vi "Application UI.vi"() -> ()   [LabVIEW 2023, in "User Interface.lvlib"]
uses:
  User Interface.lvlib
  Controls/main consumer cluster.ctl
  File Classes/File/File.lvclass
  Controls/configuration cluster.ctl
  File Classes/Controls/exif data cluster.ctl
  File Classes/Controls/rename type enum.ctl
  Controls/app operation state enum.ctl
  Controls/main producer cluster.ctl
  <vilib>/Utility/error.llb/Trim Whitespace One-Sided.vi
  EXIF Modifier/EXIF UI.vi
  EXIF Modifier/EXIF Modifier.lvlib
  File Classes/File Classes.lvlib
panel:
  in  "Temp":bool
  in  "Mode":enum16{"Copy (Default)", "Move", "Rename"}(ring)
  in  "File Name Format":T1(ring)
  in  "Event Name":string
  in  "Jpg?":bool
  in  "Exclude Folder":string
  in  "Add Scanner":string
  in  "Delete Folder":bool
  in  "Add Folder":bool
  in  "Delete Scan":bool
  in  "Add Scan":bool
  in  "Exclude":i32(listbox)=-1
  in  "Scanner":i32(listbox)=-1
  in  "Log?":bool=TRUE
  in  "Pause":bool
  in  "Stop":bool
  in  "Start":bool
  out "String":string
  out "Slide":dbl(slide) scale=0.0..100.0
  in  "Destination Path":path
  in  "Source Path":path
  out "Status":string="Application started. Waiting for user input ....."
  in  "Producer Cluster In":T2
  in  "Consumer Cluster in":T3={"This VI Ref"=refnum, "Test VI"=refnum, "Q Ref"=refnum, "UE"=refnum, "Data"=variant, "Timeout"=-1, "Path List[]"=[], "Status"="", "Counter"=0, "Config"={"Source Path"=path "", "Dest Path"=path "", "Log Path"=path "", "Move?"=FALSE, "Log?"=FALSE, "Scanners"=[], "Excude Folders"=[], "Jpg?"=FALSE, "Default path"=path "", "Extended?"=FALSE, "Mode"=enum."Move", "Temp"=FALSE}, "Total"=0, "Config Path"=path "", "exif info"={"Make"="Canon\u0000", "Model"="Canon PowerShot A495\u0000", "Orientation"=0, "Date"=timestamp(0 s since 1904-01-01), "Width"=0, "Height"=0, "Square?"=FALSE, "File Name"="Canon\u0000", "Extension"="Canon\u0000", "Valid?"=FALSE, "Path"=path "", "size"=0, "No Ext?"=FALSE, "prefix?"=FALSE, "Tag"="", "Name Type"=enum."Event Sufix", "Projection Type"="Canon\u0000"}, "app operation"=enum."Start", "Log Ref"=refnum, "Start Time"=0.0, "Pause Time"=0.0, "Argument?"=FALSE, "Argument path"=path "", "Identical"=FALSE, "File.lvclass"=refnum}
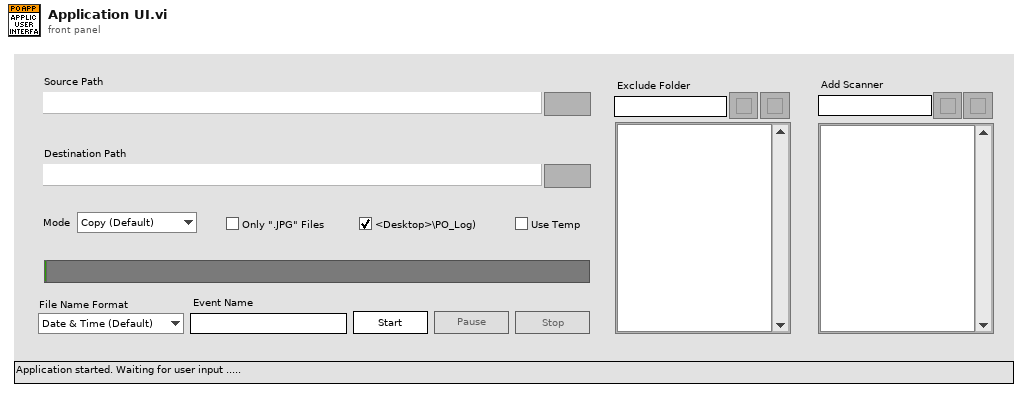
[diagram p1: front panel]
types:
  T1 = enum16{"Date & Time (Default)", "Model Sufix", "Event Sufix", "Model & Event Sufix"}
  T2 = typedef "User Interface.lvlib/main producer cluster.ctl" = cluster{"Q Ref":refnum<queue>, "menu ref":refnum<k9>, "Item Tag":string, "Is EXE?":bool, "This VI Ref":refnum<vi>, "States To Execute":string[]}
  T3 = typedef "User Interface.lvlib/main consumer cluster.ctl" = cluster{"This VI Ref":refnum<vi>, "Test VI":refnum<vi>, "Q Ref":refnum<queue>, "UE":refnum<event-registration>, "Data":variant, "Timeout":i32, "Path List[]":path[], "Status":string, "Counter":i32, "Config":T4, "Total":i32, "Config Path":path, "exif info":T5, "app operation":T7, "Log Ref":refnum<file>, "Start Time":dbl, "Pause Time":dbl, "Argument?":bool, "Argument path":path, "Identical":bool, "File.lvclass":refnum<class "File.lvclass">}
  T4 = typedef "User Interface.lvlib/configuration cluster.ctl" = cluster{"Source Path":path, "Dest Path":path, "Log Path":path, "Move?":bool, "Log?":bool, "Scanners":string[], "Excude Folders":string[], "Jpg?":bool, "Default path":path, "Extended?":bool, "Mode":enum16{"Copy (Default)", "Move", "Rename"}, "Temp":bool}
  T5 = typedef "File Classes.lvlib/exif data cluster.ctl" = cluster{"Make":string, "Model":string, "Orientation":u16, "Date":timestamp, "Width":u16, "Height":u16, "Square?":bool, "File Name":string, "Extension":string, "Valid?":bool, "Path":path, "size":i64, "No Ext?":bool, "prefix?":bool, "Tag":string, "Name Type":T6, "Projection Type":string}
  T6 = typedef "File Classes.lvlib/rename type enum.ctl" = enum16{"Date & Time (Default)", "Model Sufix", "Event Sufix", "Model & Event Sufix"}
  T7 = typedef "User Interface.lvlib/app operation state enum.ctl" = enum16{"Start", "Stop", "Pause", "Resume"}
  T8 = enum32{"invalid app kind", "Development System", "Run Time System", "Student Edition", "Embedded LabVIEW", "Evaluation", "Custom"}
  T9 = enum8{"Enabled", "Disabled", "Disabled and Grayed Out"}
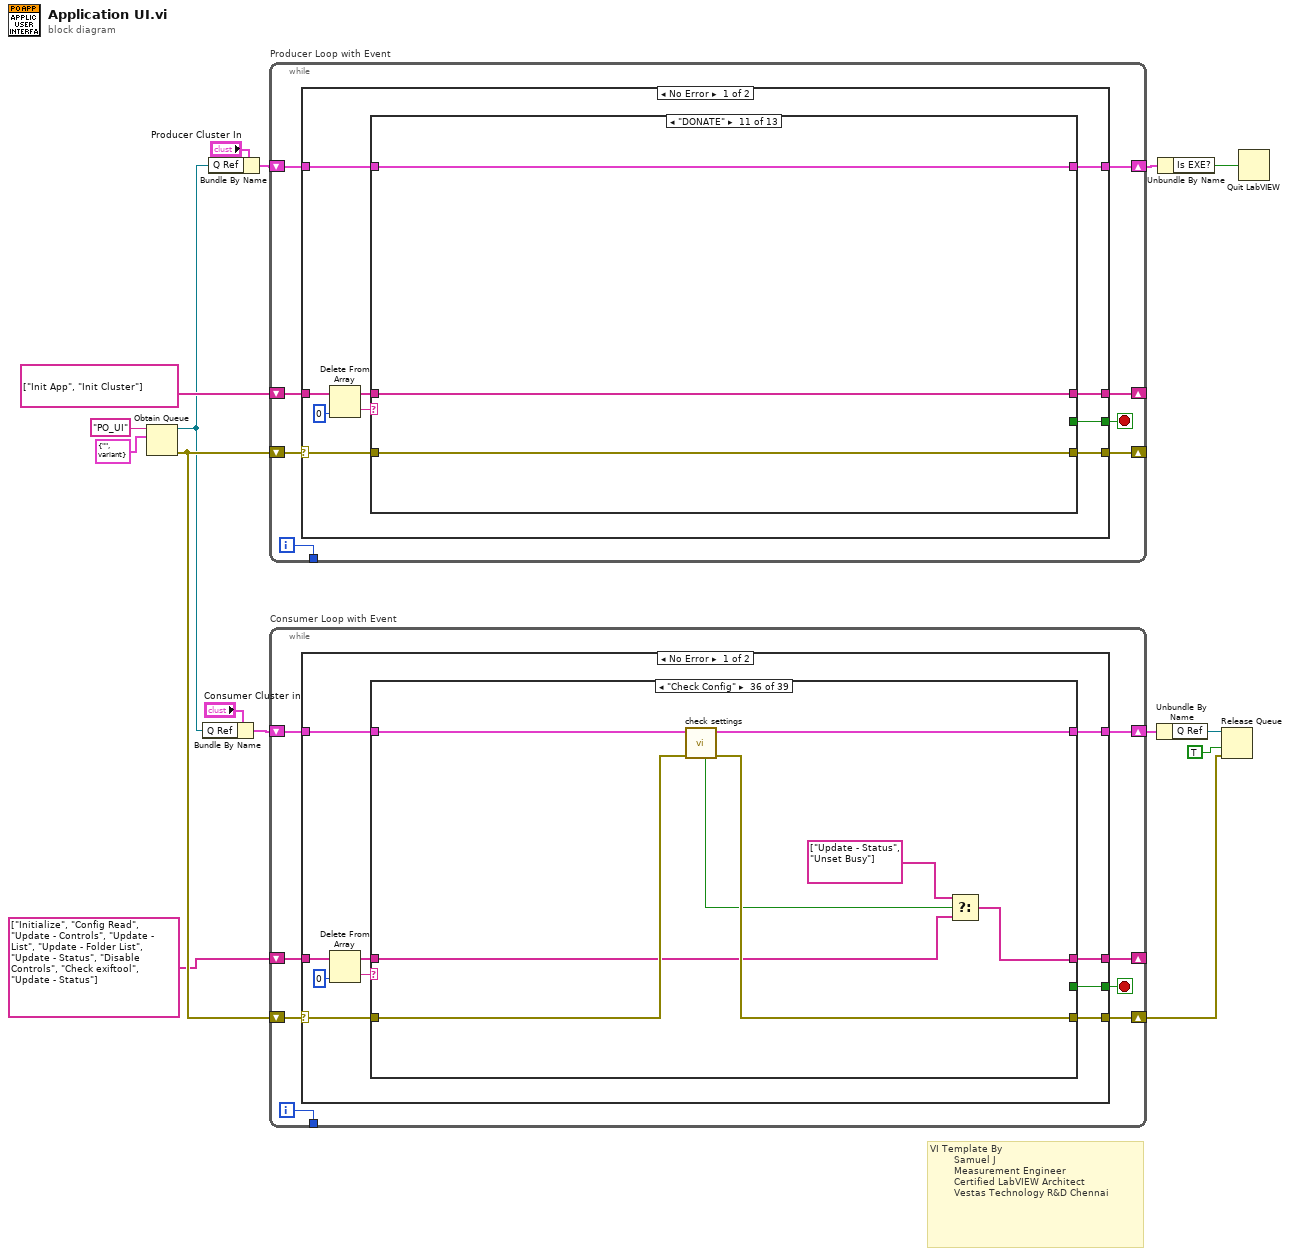
[diagram p0: block diagram]
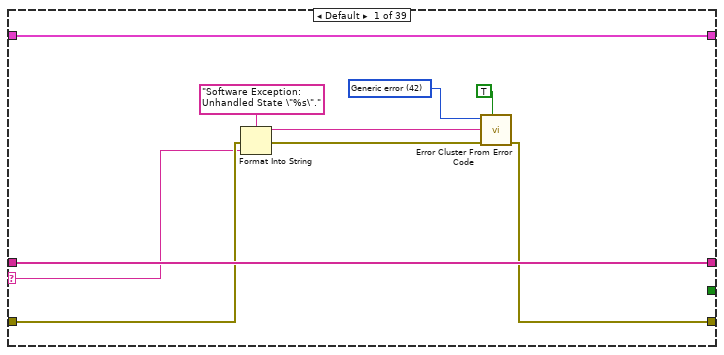
[diagram p2: hidden frame]
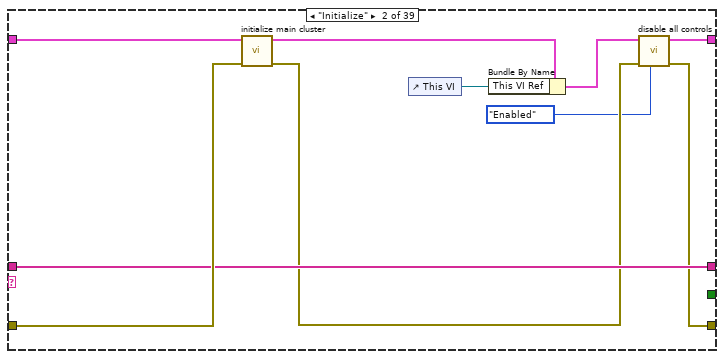
[diagram p3: hidden frame]
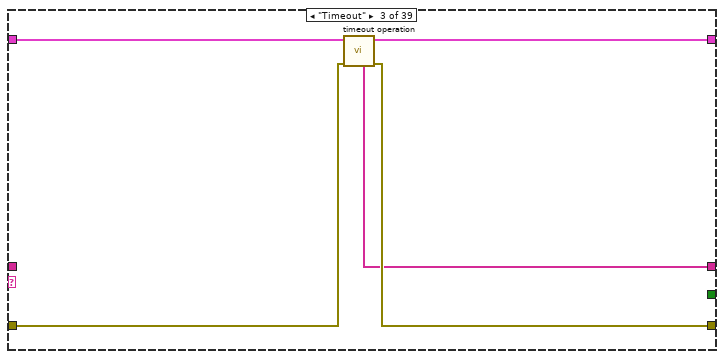
[diagram p4: hidden frame]
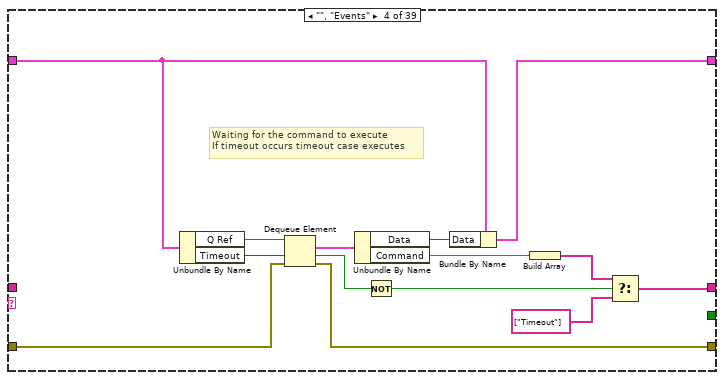
[diagram p5: hidden frame]
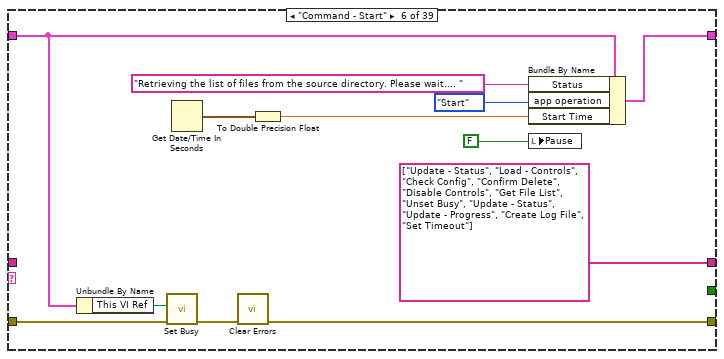
[diagram p7: hidden frame]
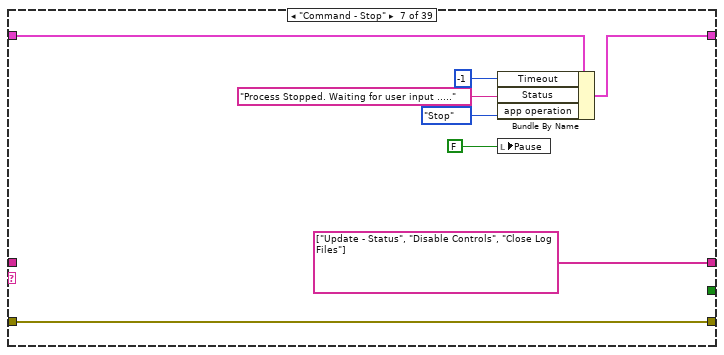
[diagram p8: hidden frame]
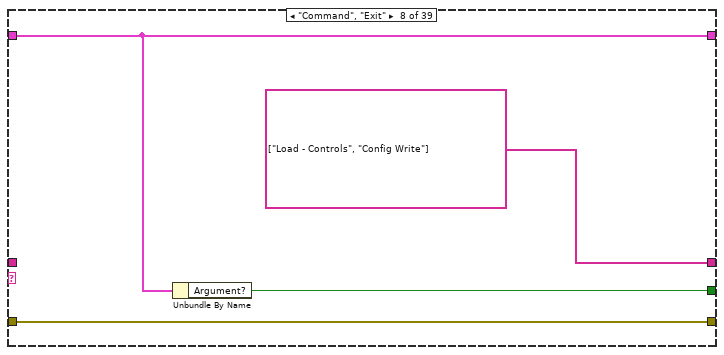
[diagram p9: hidden frame]
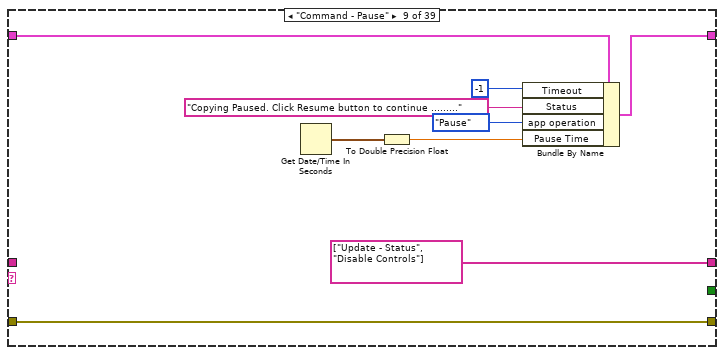
[diagram p10: hidden frame]
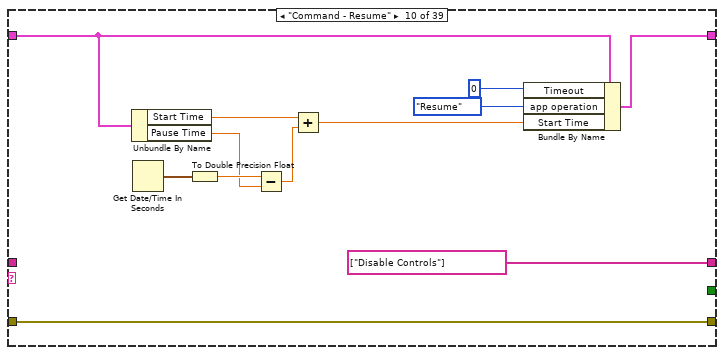
[diagram p11: hidden frame]
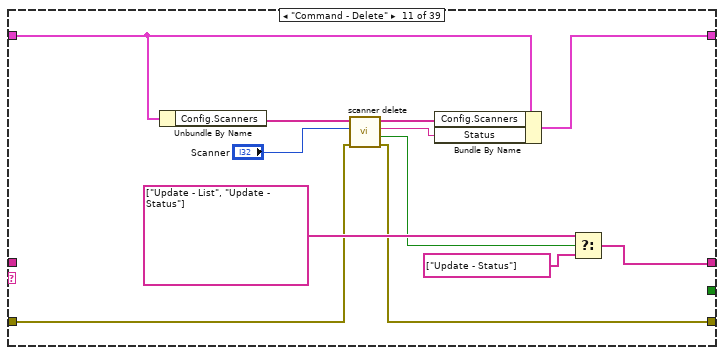
[diagram p12: hidden frame]
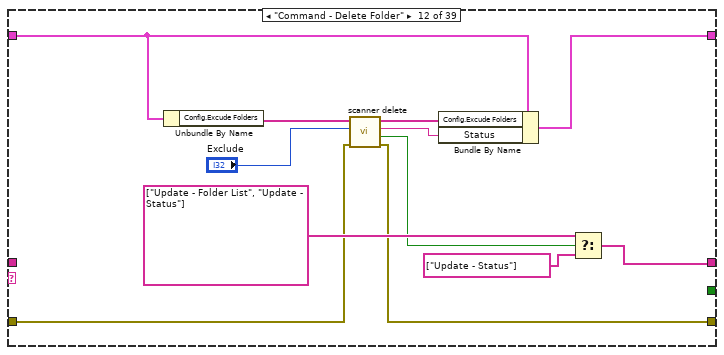
[diagram p13: hidden frame]
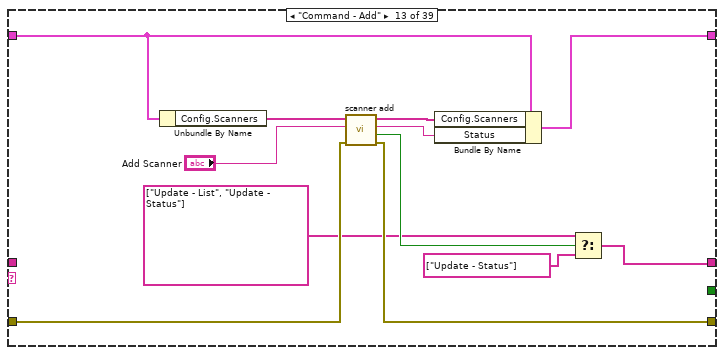
[diagram p14: hidden frame]
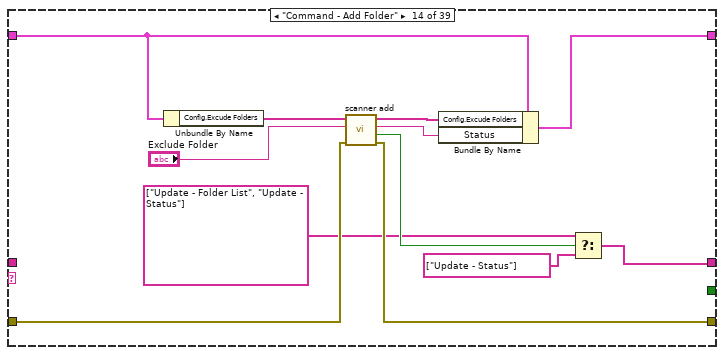
[diagram p15: hidden frame]
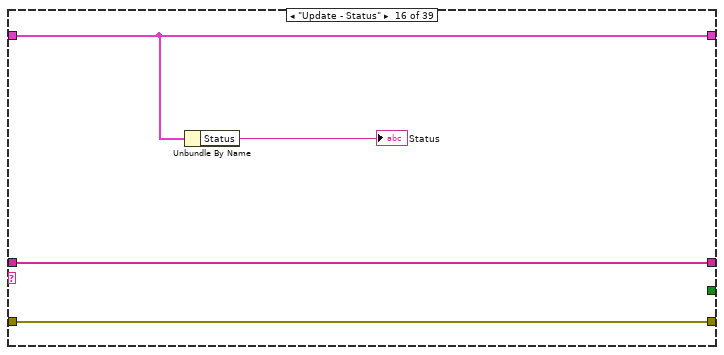
[diagram p17: hidden frame]
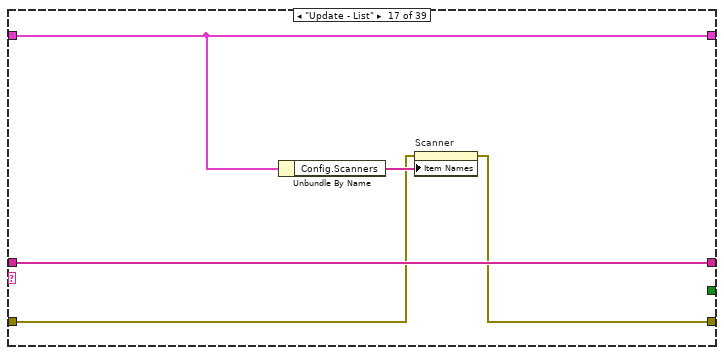
[diagram p18: hidden frame]
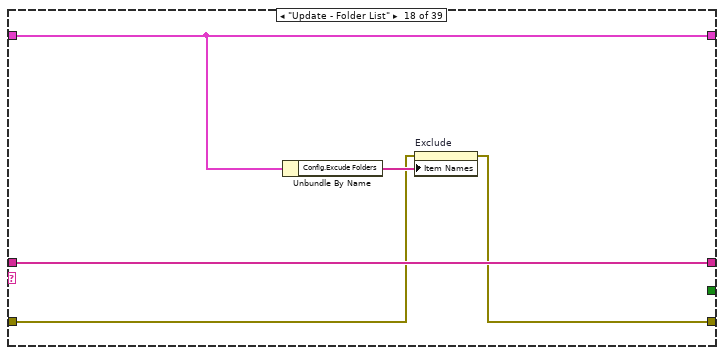
[diagram p19: hidden frame]
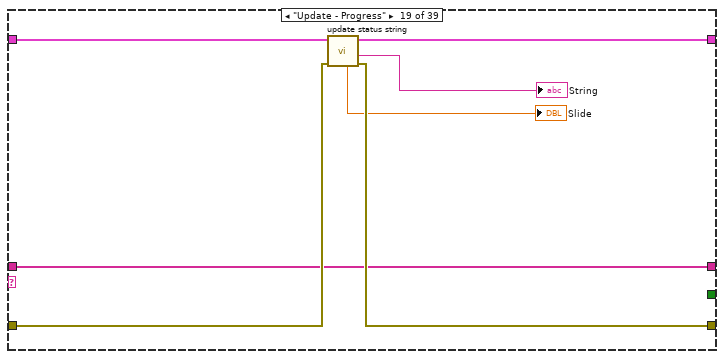
[diagram p20: hidden frame]
diagram:
  # "VI Template By\n        Samuel J\n        Measurement Engineer\n        Certified LabVIEW Architect\n        Vestas Technology R&D Chennai"
  n1 = Obtain Queue(name (unnamed)="PO_UI", element data type=cluster{"Command":string, "Data":variant} {"Command"="", "Data"=variant} ("Data Cluster")) -> (queue out=w12:refnum<queue>, error out=w13:errorcluster)  [unwired: 3 in, 1 out]
  n2 = Bundle By Name(cluster="Consumer Cluster in", "Q Ref"=w12) -> (w14:T3)
  n3 = Bundle By Name(cluster="Producer Cluster In", "Q Ref"=w12) -> (w7:T2)
  n4 = while "Producer Loop with Event" {
    shift-right: [w23] -> _
    shift-left: w13 -> [w24]
    shift-right: [w20] -> _
    shift-left: string[] ["Init App", "Init Cluster"] ("appended array") -> [w21]
    shift-right: [w18] -> w8
    shift-left: w7 -> [w19]
    tunnel: [w17] -> _
    i -> [w17]
    stop <- w22 stop-if-true
    n5 = case shown="No Error" w24 {
      selector: w24 -> [w34 w207]
      tunnel: [w33 w211] -> w23
      tunnel: [w32 FALSE] -> w22
      tunnel: w21 -> [w31 _]
      tunnel: [w27 string[] []] -> w20
      tunnel: w19 -> [w26 w206]
      tunnel: [w25 w206] -> w18
      frame No Error {
        n6 = Delete From Array(array=w31, index=0) -> (deleted portion=w29:string, array with subset deleted=w28:string[])  [unwired: 1 in]
        n7 = case shown="\"DONATE\"" w29 {
          selector: w29 -> [w37 _ _ _ _ _ _ _ _ _ _ _ _]
          tunnel: w34 -> [w39 w56 w65 w70 w86 w162 w167 w177 w185 w189 w192 w195 w199]
          tunnel: [w38 w49 w65 w68 w85 w162 w167 w178 w185 w189 w192 w195 w198] -> w33
          tunnel: [FALSE FALSE _ FALSE ("T button?") FALSE ("T button?") _ _ _ FALSE _ _ _ TRUE ("T button?")] -> w32
          tunnel: w28 -> [w45 w61 w64 w73 w84 w161 _ w180 w186 w188 w191 w194 w204]
          tunnel: [w45 w61 w64 w73 w83 w161 string[] ["Enqueue"] w180 w186 w188 w191 w194 w204] -> w27
          tunnel: w26 -> [w36 w62 w63 w71 w81 w160 w163 w179 w182 w187 w190 w193 w202]
          tunnel: [w36 w59 w63 w71 w82 w160 w164 w179 w182 w187 w190 w193 w202] -> w25
          frame Default {
            w41 = 42 items=["No error", "Argument error", "Memory is full", "Out of zone", "End of file", "File already open", "Generic file I/O error", "File not found", "File permission error", "Disk is full", "Duplicate path", "Too many files open", "System feature not enabled", "Resource file not found", "Cannot add resource", "Resource not found", "Image not found", "Image memory error", "Pen does not exist", "Config type invalid", "Config token not found", "Config parse error", "Config memory error", "Bad external code format", "Bad external code offset", "External code not present", "Null window", "Destroy window error", "Null menu", "Print aborted", "Bad print record", "Print driver error", "Windows error during printing", "Memory error during printing", "Print dialog error", "Generic print error", "Invalid device refnum", "Device not found", "Device parameter error", "Device unit error", "Cannot open device", "Device call aborted", "Generic error", "Cancelled by user", "Object ID too low", "Object ID too high", "Object not in heap", "Unknown heap", "Unknown object (invalid DefProc)", "Unknown object (DefProc not in table)", "Message out of range", "Invalid (null) method", "Unknown message", "Manager call not supported", "Bad address", "Network operation in progress", "Network operation timed out", "Connection is busy", "Network attribute not supported", "Network error", "Address in use", "System out of memory", "Connection aborted", "Connection refused", "Not connected", "Already connected", "Connection closed", "Initialization error (interapplication manager)", "Bad occurrence", "Wait on unbound occurrence handler", "Occurrence queue overflow", "Datalog type conflict", "Unused", "Unrecognized type (interapplication manager)", "Memory corrupt", "Failed to make temporary DLL", "Old CIN version", "Drag socket not found", "Failed to load drop-object", "Failed to register OLE object", "Failed to release OLE object", "Format specifier type mismatch", "Unknown format specifier", "Too few format specifiers", "Too many format specifiers", "Scan failed", "Newer CIN version", "Error converting to variant", "Runtime menu error", "Password tampered", "Variant attribute not found", "Incompatible variant data type", "Event data is not available", "Event Store is not present", "Occurrence is not found", "Event Queue is not created", "Event info is not available", "Refnum passed is NULL", "Error retrieving Class GUID", "Error retrieving CoClass GUID", "Error retrieving TypeLib GUID.", "Bad built application magic bytes.", "Specific driver is different from the specific driver associated with the Logical Name.", "There is no session opened to the class driver.", "Max Error", "MAX - Error with config objects", "MAX - Error loading configuration", "MAX - Group not supported"]
            n8 = Format Into String(format string="Software Exception: Unhandled State \"%s\"." ("message"), error in=w39, w37) -> (resulting string=w42:string, error out=w43:errorcluster)  [unwired: 1 in]
            n9 = call <vilib>:"Error Cluster From Error Code.vi"("show call chain? (False)"=TRUE, "error in (no error)"=w43, "error message (\"\")"=w42, "error code (0)"=w41) -> ("error out"=w38:errorcluster)  [unwired: 5 out]
          }
          frame "Init App" {
            n10 = property class="App"(error in=w56) -> (error out=w52:errorcluster, "App.Kind"=w54:T8)  [unwired: 1 in, 1 out]
            n11 = control-ref of="This VI"() -> (w57:refnum<vi>)
            n12 = Equal?(x=w54, y=T8."Run Time System" ("Application:Kind")) -> (x = y?=w53:bool)
            n13 = Current VI's Menubar() -> (w58:refnum<k9>)
            n14 = call <userlib>:"Set Pane Orgin 00.vi"("error in"=w52) -> ("error out"=w47:errorcluster)  [unwired: 10 in]
            n15 = Bundle By Name(cluster=w62, "menu ref"=w58, "This VI Ref"=w57, "Is EXE?"=w53) -> (w59:T2)
            n16 = call "get version info.vi"("error in"=w47) -> ("error out"=w46:errorcluster, "Title"=w48:string)  [unwired: 8 in, 1 out]
            n17 = property class="VI"(error in=w46, "Front Panel.Title"=w48) -> (error out=w49:errorcluster)  [unwired: 1 in, 1 out]
            n18 = local write "File Name Format"(T1."Model Sufix" ("File Name Format")) -> ()
            n19 = property on="Mode" class="Enum (strict)"("Val(Sgnl)"=enum16{"Copy (Default)", "Move", "Rename"}."Copy (Default)" ("Mode")) -> ()  [unwired: 2 in, 2 out]
          }
          frame "Init Cluster" {
          }
          frame "Enqueue" {
            n20 = Unbundle By Name(w71) -> ("Q Ref"=w69:refnum<queue>, "States To Execute"=w67:string[])
            n21 = for {
              tunnel: w69 -> [w78]
              shift-right: [w77] -> w68
              shift-left: w70 -> [w79]
              tunnel: w67 -> [w76] mode=indexing
              tunnel: variant ("Data") -> [w75]
              n22 = Bundle("element"=w76, "Data"=w75) -> (w74:cluster{"element":string, "Data":variant})  [unwired: 1 in]
              n23 = Enqueue Element(queue=w78, element=w74, error in (no error)=w79) -> (error out=w77:errorcluster)  [unwired: 1 in, 2 out]
            }
          }
          frame "", "Events" {
            n24 = event shown="[3] \"Start\": Value Change" {
              selector: _ -> [_ _ _ _ _ _ _ _ _ _ _ _]
              dyn-events: _ -> [_ _ _ _ _ _ _ _ _ _ _ _]
              timeout: _ -> [_ _ _ _ _ _ _ _ _ _ _ _]
              tunnel: w86 -> [w90 w93 w97 w102 w110 w117 w122 w127 w132 w137 w145 w157]
              tunnel: [w90 w93 w97 w102 w109 w117 w122 w127 w132 w137 w145 w157] -> w85
              tunnel: w84 -> [_ _ _ _ w112 _ _ _ _ _ _ w147]
              tunnel: [string[] ["EXIT"] string[] [] w94 string[] ["Enqueue"] w112 string[] ["Enqueue"] string[] ["Enqueue"] string[] ["Enqueue"] string[] ["Enqueue"] string[] ["Enqueue"] string[] ["Enqueue"] w150] -> w83
              tunnel: [w89 w92 w96 w99 w111 w114 w119 w124 w129 w134 w142 w151] -> w82
              tunnel: w81 -> [w89 w92 w96 w100 w111 w115 w120 w125 w130 w135 w143 w152]
              event Panel Close? {
                n25 = event-data() -> ()  [unwired: 2 out]
                n26 = event-data("Discard?"=TRUE) -> ()  [unwired: 1 in, 1 out]
              }
              event Timeout {
                n27 = event-data() -> ()  [unwired: 2 out]
              }
              event Menu Selection (User) {
                n28 = event-data() -> ("ItemTag"=w95:string)  [unwired: 1 out]
                n29 = Build Array(w95) -> (w94:string[])
              }
              event "Start": Value Change {
                n30 = event-data() -> ()  [unwired: 2 out]
                n31 = Bundle By Name(cluster=w100, "States To Execute"=string[] ["Command - Start"]) -> (w99:T2)
              }
              event "Mode": Value Change {
                n32 = event-data() -> ("NewVal"=w107:enum16{"Copy (Default)", "Move", "Rename"})  [unwired: 1 out]
                n33 = Equal?(x=w107, y=enum16{"Copy (Default)", "Move", "Rename"}."Rename" ("NewVal")) -> (x = y?=w105:bool)
                n34 = Select(t=T9."Disabled and Grayed Out", s=w105, f=T9."Enabled" ("Disabled")) -> (s? t:f=w104:T9)
                n35 = property on="Destination Path" class="Path"(error in=w110, "DisabledEnum"=w104) -> (error out=w109:errorcluster)  [unwired: 1 in, 1 out]
              }
              event "Stop": Value Change {
                n36 = event-data() -> ()  [unwired: 2 out]
                n37 = Bundle By Name(cluster=w115, "States To Execute"=string[] ["Command - Stop"]) -> (w114:T2)
              }
              event "Add Scan": Value Change {
                n38 = event-data() -> ()  [unwired: 2 out]
                n39 = Bundle By Name(cluster=w120, "States To Execute"=string[] ["Command - Add"]) -> (w119:T2)
              }
              event "Add Folder": Value Change {
                n40 = event-data() -> ()  [unwired: 2 out]
                n41 = Bundle By Name(cluster=w125, "States To Execute"=string[] ["Command - Add Folder"]) -> (w124:T2)
              }
              event "Delete Folder": Value Change {
                n42 = event-data() -> ()  [unwired: 2 out]
                n43 = Bundle By Name(cluster=w130, "States To Execute"=string[] ["Command - Delete Folder"]) -> (w129:T2)
              }
              event "Delete Scan": Value Change {
                n44 = event-data() -> ()  [unwired: 2 out]
                n45 = Bundle By Name(cluster=w135, "States To Execute"=string[] ["Command - Delete"]) -> (w134:T2)
              }
              event "Pause": Value Change {
                n46 = event-data() -> ("NewVal"=w141:bool)  [unwired: 1 out]
                n47 = Select(t=string[] ["Command - Pause"], s=w141, f=string[] ["Command - Resume"]) -> (s? t:f=w139:string[])
                n48 = Bundle By Name(cluster=w143, "States To Execute"=w139) -> (w142:T2)
              }
              event Key Down {
                n49 = event-data() -> ("Char"=w156:i16, "PlatMods.Ctrl"=w154:bool, "PlatMods.Alt"=w153:bool)  [unwired: 4 out]
                n50 = Or(x=w154, y=w153) -> (x .or. y?=w148:bool)
                n51 = Boolean To (0,1)(Boolean=w148) -> (0, 1=w155:i16)
                n52 = Multiply(x=w156, y=w155) -> (x*y=w146:i16)
                n53 = case shown="111" w146 {
                  tunnel: [w158 string[] ["Enqueue"]] -> w150
                  tunnel: w147 -> [w158 _]
                  frame Default {
                  }
                  frame 111 {
                  }
                }
                n54 = Bundle By Name(cluster=w152, "States To Execute"=string[] ["Option - GUI"]) -> (w151:T2)
              }
            }
          }
          frame "--------- EVENTS ---------" {
            # "Don't delete this case\nTo add a event case duplicate this case and add case selector"
          }
          frame "CONFIGURATION" {
            n55 = Bundle By Name(cluster=w163, "States To Execute"=string[] ["Option - GUI"]) -> (w164:T2)
          }
          frame "EXIF EDITOR" {
            # "0x01 Record modifications \n0x02 Open templates for editing\n0x04 Prompt user to save \n0x08 Prepare for reentrant run \n0x10 Prompt to find missing subVIs \n0x20 Hide loading dialog box\n0x40 Enable simultaneous calls on reentrant VIs  \n0x80 Prepare to call and forget \n0x100 Prepare to call and collect"
            n56 = vi-ref "EXIF Modifier.lvlib:EXIF UI.vi"() -> (w176:refnum<vi>)
            n57 = property class="VI Interface Type 0"(reference=w176, error in=w177) -> (reference out=w169:refnum<vi>, error out=w173:errorcluster, "Path"=w168:path)
            n58 = Open VI Reference(type specifier VI Refnum (for type only)=w169, vi path=w168, options=128, error in (no error)=w173) -> (vi reference=w175:refnum<vi>, error out=w172:errorcluster)  [unwired: 2 in]
            n59 = call-by-ref "Start Asynchronous Call"(reference=w175, error in=w172) -> (reference out=w174:refnum<vi>, error out=w171:errorcluster)  [unwired: 12 in]
            n60 = Close Reference(reference=w174, error in (no error)=w171) -> (error out=w178:errorcluster)
          }
          frame "CONTEXT_HELP" {
            # "Toggle Show/Hide Context Help Window"
            n61 = fn#1354() -> (1:w183:bool)  [unwired: 1 out]
            n62 = Not(x=w183) -> (.not. x?=w184:bool)
            n63 = Control Help Window(1:w184) -> ()  [unwired: 1 out]
          }
          frame "HELP" {
          }
          frame "DONATE" {
          }
          frame "ABOUT" {
          }
          frame "EXIT" {
            n64 = Unbundle By Name(w202) -> ("This VI Ref"=w200:refnum<vi>, "Is EXE?"=w201:bool, "Q Ref"=w197:refnum<queue>)
            n65 = case shown="True" w201 {
              tunnel: w200 -> [_ w205]
              frame False {
              }
              frame True {
                n66 = invoke class="VI" method="FP.Close"(reference=w205) -> ()  [unwired: 2 in, 3 out]
              }
            }
            n67 = Enqueue Element(queue=w197, element=cluster{"Command":string, "Data":variant} {"Command"="Exit", "Data"=variant}, error in (no error)=w199) -> (error out=w198:errorcluster)  [unwired: 1 in, 2 out]
          }
        }
      }
      frame Error {
        n68 = Unbundle By Name(w207) -> ("code"=w208:i32)
        n69 = case shown="42" w208 {
          tunnel: [w213 w215] -> w212
          tunnel: w207 -> [w213 w214]
          frame Default {
          }
          frame 42 {
            # "State Error"
            n70 = call <vilib>:"Simple Error Handler.vi"("error in (no error)"=w214) -> ("error out"=w215:errorcluster)  [unwired: 1 in, 7 out]
          }
        }
        n71 = call <vilib>:"Clear Errors.vi"("error in (no error)"=w212) -> ("error out"=w211:errorcluster)  [unwired: 1 in, 5 out]
      }
    }
  }
  n72 = while "Consumer Loop with Event" {
    shift-right: [w222] -> w2
    shift-left: w13 -> [w223]
    shift-right: [w219] -> _
    shift-left: string[] ["Initialize", "Config Read", "Update - Controls", "Update - List", "Update - Folder List", "Update - Status", "Disable Controls", "Check exiftool", "Update - Status"] ("appended array") -> [w220]
    shift-right: [w216] -> w1
    shift-left: w14 -> [w218]
    tunnel: [w217] -> _
    i -> [w217]
    stop <- w221 stop-if-true
    n73 = case shown="No Error" w223 {
      selector: w223 -> [w233 w561]
      tunnel: [w232 w563] -> w222
      tunnel: [w224 w558] -> w221
      tunnel: w220 -> [w231 _]
      tunnel: [w227 string[] ["Unset Busy", "Update - Status"]] -> w219
      tunnel: w218 -> [w226 w557]
      tunnel: [w225 w555] -> w216
      frame No Error {
        n74 = Delete From Array(array=w231, index=0) -> (deleted portion=w229:string, array with subset deleted=w228:string[])  [unwired: 1 in]
        n75 = case shown="\"Check Config\"" w229 {
          selector: w229 -> [w235 _ _ _ _ _ _ _ _ _ _ _ _ _ _ _ _ _ _ _ _ _ _ _ _ _ _ _ _ _ _ _ _ _ _ _ _ _ _]
          tunnel: w233 -> [w237 w253 w255 w271 w275 w284 w295 w299 w308 w320 w323 w336 w354 w367 w371 w375 w377 w382 w392 w405 w412 w417 w422 w433 w448 w454 w457 w461 w471 w478 w482 w494 w501 w505 w524 w528 w537 w546 w552]
          tunnel: [w236 w246 w256 w270 w275 w276 w295 w299 w308 w320 w322 w335 w353 w366 w371 w375 w376 w381 w389 w405 w412 w418 w423 w433 w446 w453 w456 w461 w467 w478 w481 w493 w498 w504 w524 w527 w537 w545 w551] -> w232
          tunnel: w228 -> [w243 w252 _ _ w274 _ _ _ _ _ _ _ _ _ w370 w374 w380 w385 w386 w404 w411 w414 w426 w432 w450 w455 w460 w466 w472 w477 w484 w497 w503 w508 w523 w525 w534 w549 w550]
          tunnel: [w243 w252 w254 w262 w274 string[] ["Update - Status", "Load - Controls", "Check Config", "Confirm Delete", "Disable Controls", "Get File List", "Unset Busy", "Update - Status", "Update - Progress", "Create Log File", "Set Timeout"] ("f") string[] ["Update - Status", "Disable Controls", "Close Log Files"] ("appended array") string[] ["Load - Controls", "Config Write"] ("appended array") string[] ["Update - Status", "Disable Controls"] ("f") string[] ["Disable Controls"] ("appended array") w330 w342 w347 w360 w370 w374 w380 w385 w386 w404 w411 w415 w426 w432 w450 w455 w460 w466 w472 w477 w484 w497 w503 w508 w523 w532 w533 w549 w550] -> w227
          tunnel: w226 -> [w234 w249 w258 w268 w273 w282 w294 w297 w307 w315 w332 w344 w351 w364 w369 w373 w379 w384 w390 w403 w410 w420 w425 w431 w449 w452 w459 w462 w469 w476 w480 w496 w502 w507 w519 w530 w536 w548 w553]
          tunnel: [w234 w248 w257 w267 w273 w286 w293 w297 w306 w319 w331 w343 w350 w363 w369 w373 w379 w384 w391 w403 w410 w419 w424 w431 w447 w452 w458 w465 w469 w475 w483 w495 w499 w506 w522 w529 w536 w547 w554] -> w225
          tunnel: [_ _ _ _ _ _ _ w296 _ _ _ _ _ _ _ _ _ _ _ _ _ _ _ _ _ _ _ _ _ _ _ TRUE _ _ _ _ _ _ _] -> w224
          frame Default {
            w239 = 42 items=["No error", "Argument error", "Memory is full", "Out of zone", "End of file", "File already open", "Generic file I/O error", "File not found", "File permission error", "Disk is full", "Duplicate path", "Too many files open", "System feature not enabled", "Resource file not found", "Cannot add resource", "Resource not found", "Image not found", "Image memory error", "Pen does not exist", "Config type invalid", "Config token not found", "Config parse error", "Config memory error", "Bad external code format", "Bad external code offset", "External code not present", "Null window", "Destroy window error", "Null menu", "Print aborted", "Bad print record", "Print driver error", "Windows error during printing", "Memory error during printing", "Print dialog error", "Generic print error", "Invalid device refnum", "Device not found", "Device parameter error", "Device unit error", "Cannot open device", "Device call aborted", "Generic error", "Cancelled by user", "Object ID too low", "Object ID too high", "Object not in heap", "Unknown heap", "Unknown object (invalid DefProc)", "Unknown object (DefProc not in table)", "Message out of range", "Invalid (null) method", "Unknown message", "Manager call not supported", "Bad address", "Network operation in progress", "Network operation timed out", "Connection is busy", "Network attribute not supported", "Network error", "Address in use", "System out of memory", "Connection aborted", "Connection refused", "Not connected", "Already connected", "Connection closed", "Initialization error (interapplication manager)", "Bad occurrence", "Wait on unbound occurrence handler", "Occurrence queue overflow", "Datalog type conflict", "Unused", "Unrecognized type (interapplication manager)", "Memory corrupt", "Failed to make temporary DLL", "Old CIN version", "Drag socket not found", "Failed to load drop-object", "Failed to register OLE object", "Failed to release OLE object", "Format specifier type mismatch", "Unknown format specifier", "Too few format specifiers", "Too many format specifiers", "Scan failed", "Newer CIN version", "Error converting to variant", "Runtime menu error", "Password tampered", "Variant attribute not found", "Incompatible variant data type", "Event data is not available", "Event Store is not present", "Occurrence is not found", "Event Queue is not created", "Event info is not available", "Refnum passed is NULL", "Error retrieving Class GUID", "Error retrieving CoClass GUID", "Error retrieving TypeLib GUID.", "Bad built application magic bytes.", "Specific driver is different from the specific driver associated with the Logical Name.", "There is no session opened to the class driver.", "Max Error", "MAX - Error with config objects", "MAX - Error loading configuration", "MAX - Group not supported"]
            n76 = Format Into String(format string="Software Exception: Unhandled State \"%s\"." ("message"), error in=w237, w235) -> (resulting string=w240:string, error out=w241:errorcluster)  [unwired: 1 in]
            n77 = call <vilib>:"Error Cluster From Error Code.vi"("show call chain? (False)"=TRUE, "error in (no error)"=w241, "error message (\"\")"=w240, "error code (0)"=w239) -> ("error out"=w236:errorcluster)  [unwired: 5 out]
          }
          frame "Initialize" {
            n78 = call "initialize main cluster.vi"("error in"=w253, "Cluster in"=w249) -> ("error out"=w245:errorcluster, "Cluster out"=w251:T3)  [unwired: 8 in]
            n79 = control-ref of="This VI"() -> (w250:refnum<vi>)
            n80 = Bundle By Name(cluster=w251, "This VI Ref"=w250) -> (w247:T3)
            n81 = call "disable all controls.vi"("DisabledEnum"=T9."Enabled", "error in"=w245, "Cluster in"=w247) -> ("error out"=w246:errorcluster, "Cluster out"=w248:T3)  [unwired: 7 in]
          }
          frame "Timeout" {
            n82 = call "timeout operation.vi"("error in"=w255, "cluster in"=w258) -> ("error out"=w256:errorcluster, "cluster out"=w257:T3, "next states[]"=w254:string[])  [unwired: 7 in]
          }
          frame "", "Events" {
            # "Waiting for the command to execute\nIf timeout occurs timeout case executes"
            n83 = Unbundle By Name(w268) -> ("Q Ref"=w272:refnum<queue>, "Timeout"=w266:i32)
            n84 = Dequeue Element(queue=w272, timeout in ms (-1)=w266, error in (no error)=w271) -> (element=w269:cluster{"Command":string, "Data":variant}, timed out?=w263:bool, error out=w270:errorcluster)  [unwired: 1 out]
            n85 = Unbundle By Name(w269) -> ("Data"=w264:variant, "Command"=w265:string)
            n86 = Not(x=w263) -> (.not. x?=w260:bool)
            n87 = Bundle By Name(cluster=w268, "Data"=w264) -> (w267:T3)
            n88 = Build Array(w265) -> (w261:string[])
            n89 = Select(t=w261, s=w260, f=string[] ["Timeout"]) -> (s? t:f=w262:string[])
          }
          frame "--------- COMMAND ---------" {
          }
          frame "Command - Start" {
            n90 = Unbundle By Name(w282) -> ("This VI Ref"=w281:refnum<vi>)
            n91 = call <vilib>:"Set Busy.vi"("error in (no error)"=w284, "VI reference (current VI)"=w281) -> ("error out"=w283:errorcluster)  [unwired: 8 in, 1 out]
            n92 = Get Date/Time In Seconds() -> (seconds since 1Jan1904=w279:timestamp)
            n93 = call <vilib>:"Clear Errors.vi"("error in (no error)"=w283) -> ("error out"=w276:errorcluster)  [unwired: 5 in, 1 out]
            n94 = To Double Precision Float(number=w279) -> (double precision float=w278:dbl)
            n95 = Bundle By Name(cluster=w282, "Status"="Retrieving the list of files from the source directory. Please wait.... ", "app operation"=app_operation_state_enum."Start" ("Enum"), "Start Time"=w278) -> (w286:T3)
            n96 = local write "Pause"(FALSE ("Pause")) -> ()
          }
          frame "Command - Stop" {
            n97 = Bundle By Name(cluster=w294, "Timeout"=-1, "Status"="Process Stopped. Waiting for user input .....", "app operation"=app_operation_state_enum."Stop" ("Enum")) -> (w293:T3)
            n98 = local write "Pause"(FALSE ("Pause")) -> ()
          }
          frame "Command", "Exit" {
            n99 = Unbundle By Name(w297) -> ("Argument?"=w296:bool)
          }
          frame "Command - Pause" {
            n100 = Get Date/Time In Seconds() -> (seconds since 1Jan1904=w301:timestamp)
            n101 = To Double Precision Float(number=w301) -> (double precision float=w300:dbl)
            n102 = Bundle By Name(cluster=w307, "Timeout"=-1, "Status"="Copying Paused. Click Resume button to continue .........", "app operation"=app_operation_state_enum."Pause" ("Enum"), "Pause Time"=w300) -> (w306:T3)
          }
          frame "Command - Resume" {
            n103 = Unbundle By Name(w315) -> ("Start Time"=w310:dbl, "Pause Time"=w312:dbl)
            n104 = Get Date/Time In Seconds() -> (seconds since 1Jan1904=w314:timestamp)
            n105 = To Double Precision Float(number=w314) -> (double precision float=w313:dbl)
            n106 = Subtract(x=w313, y=w312) -> (x-y=w311:dbl)
            n107 = Add(x=w310, y=w311) -> (x+y=w309:dbl)
            n108 = Bundle By Name(cluster=w315, "Timeout"=0, "app operation"=app_operation_state_enum."Resume" ("Enum"), "Start Time"=w309) -> (w319:T3)
          }
          frame "Command - Delete" {
            n109 = Unbundle By Name(w332) -> ("Config.Scanners"=w327:string[])
            n110 = call "scanner delete.vi"("error in"=w323, "Index"="Scanner", "Config.Scanners"=w327) -> ("error out"=w322:errorcluster, "Valid"=w321:bool, "Error"=w325:string, "Config.Scanners"=w326:string[])  [unwired: 5 in]
            n111 = Bundle By Name(cluster=w332, "Config.Scanners"=w326, "Status"=w325) -> (w331:T3)
            n112 = Select(t=string[] ["Update - List", "Update - Status"] ("f"), s=w321, f=string[] ["Update - Status"]) -> (s? t:f=w330:string[])
          }
          frame "Command - Delete Folder" {
            n113 = Unbundle By Name(w344) -> ("Config.Excude Folders"=w339:string[])
            n114 = call "scanner delete.vi"("error in"=w336, "Index"="Exclude", "Config.Scanners"=w339) -> ("error out"=w335:errorcluster, "Valid"=w334:bool, "Error"=w337:string, "Config.Scanners"=w338:string[])  [unwired: 5 in]
            n115 = Bundle By Name(cluster=w344, "Config.Excude Folders"=w338, "Status"=w337) -> (w343:T3)
            n116 = Select(t=string[] ["Update - Folder List", "Update - Status"] ("f"), s=w334, f=string[] ["Update - Status"]) -> (s? t:f=w342:string[])
          }
          frame "Command - Add" {
            n117 = Unbundle By Name(w351) -> ("Config.Scanners"=w356:string[])
            n118 = call "scanner add.vi"("error in"=w354, "String"="Add Scanner", "Config.Scanners"=w356) -> ("error out"=w353:errorcluster, "Valid"=w348:bool, "Error"=w349:string, "Config.Scanners"=w352:string[])  [unwired: 5 in]
            n119 = Bundle By Name(cluster=w351, "Config.Scanners"=w352, "Status"=w349) -> (w350:T3)
            n120 = Select(t=string[] ["Update - List", "Update - Status"] ("f"), s=w348, f=string[] ["Update - Status"]) -> (s? t:f=w347:string[])
          }
          frame "Command - Add Folder" {
            n121 = Unbundle By Name(w364) -> ("Config.Excude Folders"=w368:string[])
            n122 = call "scanner add.vi"("error in"=w367, "String"="Exclude Folder", "Config.Scanners"=w368) -> ("error out"=w366:errorcluster, "Valid"=w361:bool, "Error"=w362:string, "Config.Scanners"=w365:string[])  [unwired: 5 in]
            n123 = Bundle By Name(cluster=w364, "Config.Excude Folders"=w365, "Status"=w362) -> (w363:T3)
            n124 = Select(t=string[] ["Update - Folder List", "Update - Status"] ("f"), s=w361, f=string[] ["Update - Status"]) -> (s? t:f=w360:string[])
          }
          frame "----------- UPDATE -----------" {
          }
          frame "Update - Status" {
            n125 = Unbundle By Name(w373) -> ("Status"=→"Status":string)
          }
          frame "Update - List" {
            n126 = Unbundle By Name(w379) -> ("Config.Scanners"=w378:string[])
            n127 = property on="Scanner" class="LstBox (strict)"(error in=w377, "Item Names"=w378) -> (error out=w376:errorcluster)  [unwired: 1 in, 1 out]
          }
          frame "Update - Folder List" {
            n128 = Unbundle By Name(w384) -> ("Config.Excude Folders"=w383:string[])
            n129 = property on="Exclude" class="LstBox (strict)"(error in=w382, "Item Names"=w383) -> (error out=w381:errorcluster)  [unwired: 1 in, 1 out]
          }
          frame "Update - Progress" {
            n130 = call "update status string.vi"("error in"=w392, "Consumer Cluster in"=w390) -> ("error out"=w389:errorcluster, "String"=→"String":string, "cluster out"=w391:T3, "Slide"=→"Slide":dbl)  [unwired: 6 in]
          }
          frame "Update - Controls" {
            n131 = Unbundle By Name(w403) -> ("Argument?"=w401:bool, "Argument path"=w399:path, "Config.Source Path"=w398:path, "Config.Dest Path"=w395:path, "Config.Default path"=w397:path, "Config.Temp"=w393:bool, "Config.Log?"=w402:bool, "exif info.Tag"=w394:string)  [unwired: 1 out]
            n132 = local write "Temp"(w393) -> ()
            n133 = local write "Log?"(w402) -> ()
            n134 = local write "Event Name"(w394) -> ()
            n135 = case shown="False" w401 {
              tunnel: [w407 w409] -> w400
              tunnel: w399 -> [_ w409]
              tunnel: w398 -> [w407 _]
              tunnel: w397 -> [_ w408]
              tunnel: [w406 w408] -> w396
              tunnel: w395 -> [w406 _]
              frame False {
              }
              frame True {
              }
            }
            n136 = local write "Destination Path"(w396) -> ()
            n137 = local write "Source Path"(w400) -> ()
          }
          frame "--------- OPERATIONS --------" {
          }
          frame "Check exiftool" {
            n138 = call "check exiftool.vi"("error in"=w417, "Cluster in"=w420) -> ("error out"=w418:errorcluster, "Cluster out"=w419:T3, "success?"=w416:bool)  [unwired: 7 in]
            n139 = Select(t=w414, s=w416, f=string[] ["Update - Status", "Disable All Controls"]) -> (s? t:f=w415:string[])
          }
          frame "Disable All Controls" {
            n140 = call "disable all controls.vi"("DisabledEnum"=T9."Disabled and Grayed Out", "error in"=w422, "Cluster in"=w425) -> ("error out"=w423:errorcluster, "Cluster out"=w424:T3)  [unwired: 7 in]
          }
          frame "Disable Controls" {
            n141 = Unbundle By Name(w431) -> ("app operation"=w430:T7)
            n142 = case shown="\"Resume\"" w430 {
              tunnel: [T9."Disabled and Grayed Out" ("Disabled") T9."Enabled" ("Disabled") T9."Enabled" ("Disabled") T9."Enabled" ("Disabled")] -> w429
              tunnel: [T9."Enabled" ("Disabled") T9."Disabled and Grayed Out" ("Disabled") T9."Disabled and Grayed Out" ("Disabled") T9."Disabled and Grayed Out" ("Disabled")] -> w428
              tunnel: [T9."Disabled and Grayed Out" ("Disabled") T9."Enabled" ("Disabled") T9."Enabled" ("Disabled") T9."Enabled" ("Disabled")] -> w427
              frame "Stop", Default {
              }
              frame "Pause" {
              }
              frame "Resume" {
              }
              frame "Start" {
              }
            }
            n143 = property on="Pause" class="Bool (strict)"("DisabledEnum"=w429) -> ()  [unwired: 2 in, 2 out]
            n144 = property on="Start" class="Bool"("DisabledEnum"=w428) -> ()  [unwired: 2 in, 2 out]
            n145 = property on="Stop" class="Bool"("DisabledEnum"=w427) -> ()  [unwired: 2 in, 2 out]
          }
          frame ">>>>>>1", "Picture - Process" {
            n146 = call "process selected file.vi"("error in"=w448, "Cluster in"=w449) -> ("error out"=w446:errorcluster, "Cluster out"=w447:T3)  [unwired: 8 in]
          }
          frame "Picture - Copy" {
            n147 = Unbundle By Name(w452) -> ("File.lvclass"=w451:refnum<class "File.lvclass">)
            n148 = call-dynamic "file operation.vi"("error in (no error)"=w454, "File in"=w451) -> ("error out"=w453:errorcluster)  [unwired: 8 in, 1 out]
          }
          frame "Set Updates" {
            n149 = call "log status.vi"("error in"=w457, "Cluster in"=w459) -> ("error out"=w456:errorcluster, "Cluster out"=w458:T3)  [unwired: 8 in]
          }
          frame "Process Completed" {
            n150 = Bundle By Name(cluster=w462, "Timeout"=-1, "Status"="Copied Sucessfully ... ") -> (w465:T3)
          }
          frame "Unset Busy" {
            n151 = Unbundle By Name(w469) -> ("This VI Ref"=w468:refnum<vi>)
            n152 = call <vilib>:"Unset Busy.vi"("error in (no error)"=w471, "VI reference (current VI)"=w468) -> ("error out"=w470:errorcluster)  [unwired: 9 in]
            n153 = call <vilib>:"Clear Errors.vi"("error in (no error)"=w470) -> ("error out"=w467:errorcluster)  [unwired: 5 in, 1 out]
          }
          frame "Set Timeout" {
            n154 = Bundle By Name(cluster=w476, "Counter"=-1, "Timeout"=1000) -> (w475:T3)
          }
          frame "Option - GUI" {
            n155 = Unbundle By Name(w480) -> ("Timeout"=w479:i32)
            n156 = case shown="-1" w479 {
              tunnel: w480 -> [w485 w490]
              tunnel: [w485 w489] -> w483
              tunnel: w482 -> [w486 w488]
              tunnel: [w486 w487] -> w481
              frame Default {
              }
              frame -1 {
                n157 = call "Configuration UI.vi"("error in"=w488, "Message ni"=w490) -> ("error out"=w487:errorcluster, "Message out"=w489:T3)  [unwired: 8 in]
              }
            }
          }
          frame "Config Write" {
            n158 = call "read write configuration.vi"("Enum"=enum16{"Read", "Write"}."Write", "error in"=w494, "Consumer Cluster in"=w496) -> ("error out"=w493:errorcluster, "cluster out"=w495:T3)  [unwired: 7 in]
          }
          frame "Config Read" {
            n159 = call "read write configuration.vi"("Enum"=enum16{"Read", "Write"}."Read", "error in"=w501, "Consumer Cluster in"=w502) -> ("error out"=w498:errorcluster, "cluster out"=w499:T3)  [unwired: 7 in]
          }
          frame "Get File List" {
            n160 = call "get files list.vi"("error in"=w505, "Cluster in"=w507) -> ("error out"=w504:errorcluster, "Cluster out"=w506:T3)  [unwired: 8 in]
          }
          frame "Load - Controls" {
            n161 = Unbundle By Name(w519) -> ("Config.Scanners"=w518:string[])
            n162 = call "create temp folder.vi"("Temp?"="Temp", "Path in"="Destination Path") -> ("Path out"=w509:path)  [unwired: 8 in, 1 out]
            n163 = call <vilib>:"Trim Whitespace.vi"("string"="Event Name") -> ("trimmed string"=w515:string)  [unwired: 1 in]
            n164 = Bundle By Name(cluster=w519, "Config.Temp"="Temp", "Config.Jpg?"="Jpg?", "Config.Source Path"="Source Path", "Config.Dest Path"=w509, "Config.Move?"=FALSE, "Config.Log?"="Log?", "Config.Scanners"=w518, "exif info.Name Type"="File Name Format", "exif info.Tag"=w515, "Config.Mode"="Mode") -> (w522:T3)
          }
          frame "Check Config" {
            n165 = call "check settings.vi"("error in"=w528, "cluster in"=w530) -> ("error out"=w527:errorcluster, "cluster out"=w529:T3, "Error?"=w526:bool)  [unwired: 7 in]
            n166 = Select(t=string[] ["Update - Status", "Unset Busy"], s=w526, f=w525) -> (s? t:f=w532:string[])
          }
          frame "Confirm Delete" {
            n167 = Unbundle By Name(w536) -> ("Config.Move?"=w535:bool)
            n168 = case shown="True" w535 {
              tunnel: w534 -> [w538 w541]
              tunnel: [w538 w540] -> w533
              frame False {
              }
              frame True {
                n169 = Two Button Dialog(message="You have selected \"Delete Source Files\" on copy. Please confirm?", 2:"Proceed" ("T button name (\"OK\")")) -> (T button?=w542:bool)  [unwired: 1 in]
                n170 = Select(t=w541, s=w542, f=string[] ["Unset Busy"]) -> (s? t:f=w540:string[])
              }
            }
          }
          frame "Create Log File" {
            n171 = call "create log file.vi"("error in"=w546, "Cluster in"=w548) -> ("error out"=w545:errorcluster, "Cluster out"=w547:T3)  [unwired: 8 in]
          }
          frame "Close Log Files" {
            n172 = call "close log file.vi"("error in"=w552, "Cluster in"=w553) -> ("error out"=w551:errorcluster, "Cluster out"=w554:T3)  [unwired: 8 in]
          }
        }
      }
      frame Error {
        n173 = Unbundle By Name(w561) -> ("code"=w559:i32)
        n174 = case shown="7, 1430" w559 {
          tunnel: w561 -> [w566 w571 w573 w578]
          tunnel: [w566 w570 w573 w578] -> w560
          tunnel: [TRUE FALSE FALSE FALSE] -> w558
          tunnel: w557 -> [w564 w568 w575 w580]
          tunnel: [w564 w567 w574 w579] -> w556
          frame 1, 1122 {
          }
          frame Default {
            n175 = call <vilib>:"Simple Error Handler.vi"("error in (no error)"=w571) -> ("error out"=w570:errorcluster)  [unwired: 4 in, 4 out]
            n176 = Bundle By Name(cluster=w568, "Timeout"=-1) -> (w567:T3)
          }
          frame 7, 1430 {
            n177 = Bundle By Name(cluster=w575, "Timeout"=0) -> (w574:T3)
          }
          frame 8, 1172 {
            n178 = Bundle By Name(cluster=w580, "Timeout"=0) -> (w579:T3)
          }
        }
        n179 = call "log error.vi"("error in (no error)"=w560, "Consumer Cluster in"=w556) -> ("error out"=w563:errorcluster, "Consumer Cluster in 2"=w555:T3)  [unwired: 4 in]
      }
    }
  }
  n180 = Unbundle By Name(w1) -> ("Q Ref"=w3:refnum<queue>)
  n181 = Unbundle By Name(w8) -> ("Is EXE?"=w15:bool)
  n182 = Release Queue(queue=w3, force destroy? (F)=TRUE, error in (no error)=w2) -> ()  [unwired: 3 out]
  n183 = Quit LabVIEW(quit? (T)=w15) -> ()
